vi "Set VS item parameter map.vi"(8 "error in (no error)":errorcluster, 10 "param config in":T1, 11 "Iten refs in":T5=18446744073709551615 format="%.0x") -> (0 "error out":errorcluster, 1 "Replaced":bool, 3 "Iten refs out":T5=18446744073709551615 format="%.0x")   [LabVIEW 2020, in "Ballard 1553 System Explorer.lvlib"]
uses:
  Ballard 1553 System Explorer.lvlib
  Shared/Controls and Global/Global.vi
  Shared/Ballard 1553 Shared.lvlib
  <vilib>/NI VeriStand/Custom Device API/Custom Device API.lvlib
  <vilib>/NI VeriStand/Custom Device API/Set Item Property (Variant).vi
  <vilib>/NI VeriStand/Custom Device API/Custom Device Item Ref.ctl
  Azdo/emea-ni-vscd_Configurator/source/ConfiguratorConsumer/Ballard_1553/controls/param_signalType_type.ctl
  Azdo/emea-ni-vscd_Configurator/source/ConfiguratorConsumer/Ballard_1553/Ballard_1553.lvclass
  Azdo/emea-ni-vscd_Configurator/source/ConfiguratorConsumer/Ballard_1553/controls/param_encoding_type.ctl
  Azdo/emea-ni-vscd_Configurator/source/ConfiguratorConsumer/Ballard_1553/controls/param_type.ctl
  param_map_sysdef_type.ctl
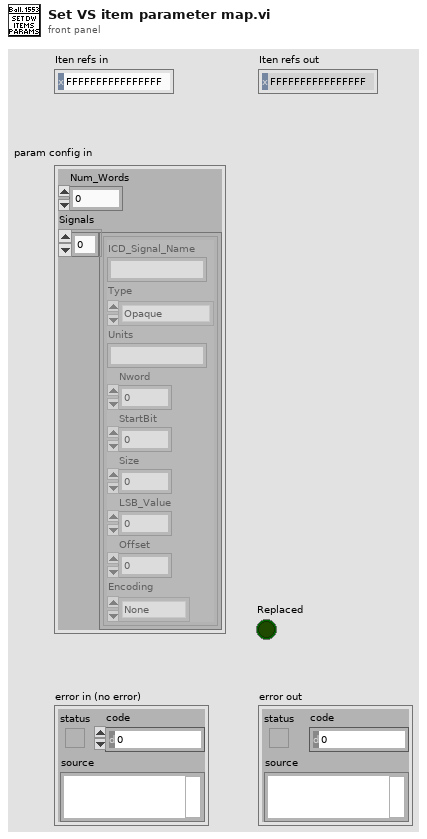
[diagram p1: front panel]
types:
  T1 = typedef "Ballard 1553 System Explorer.lvlib/param_map_sysdef_type.ctl" = cluster{"Num_Words":u8, "Signals":T2[]}
  T2 = typedef "ConfigurationManager.lvlib/Ballard_1553.lvclass/param_type.ctl" = cluster{"ICD_Signal_Name":string, "Type":T3, "Units":string, "Nword":i32, "StartBit":i32, "Size":i32, "LSB_Value":dbl, "Offset":i32, "Encoding":T4}
  T3 = typedef "ConfigurationManager.lvlib/Ballard_1553.lvclass/param_signalType_type.ctl" = enum16{"Opaque", "Enum", "Float", "Integer", "Bcd", "Bool"}
  T4 = typedef "ConfigurationManager.lvlib/Ballard_1553.lvclass/param_encoding_type.ctl" = enum16{"None", "2-complement", "Unsigned"}
  T5 = typedef "Custom Device API.lvlib/Custom Device Item Ref.ctl" = u64
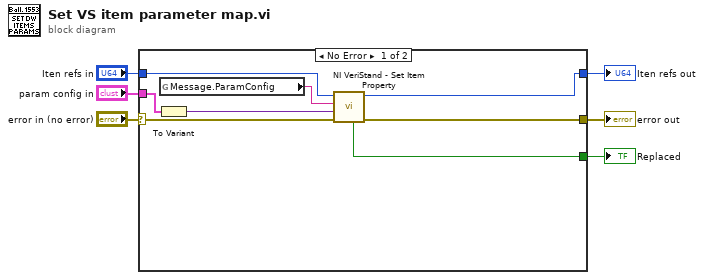
[diagram p0: block diagram]
diagram:
  n1 = case shown="No Error" "error in (no error)" {
    selector: "error in (no error)" -> [w13 w16]
    tunnel: [w10 w16] -> w5
    tunnel: [w11 w15] -> w4
    tunnel: "Iten refs in" -> [w14 w15]
    tunnel: "param config in" -> [w8 _]
    tunnel: [w9 _] -> w2
    frame No Error {
      n2 = To Variant(anything=w8) -> (Variant=w7:variant)
      n3 = global read "Global.vi" "Message.ParamConfig"() -> (w12:string)
      n4 = call-poly <vilib>:"NI VeriStand - Set Item Property.vi"("error in (no error)"=w13, "Value"=w7, "Property Name"=w12, "Item Ref in"=w14) -> ("error out"=w10:errorcluster, "Item Ref out"=w11:T5, "Replaced"=w9:bool)  [unwired: 5 in]
    }
    frame Error {
    }
  }
  "error out" <- w5
  "Iten refs out" <- w4
  "Replaced" <- w2
